vi "LoggerRefnumGetSet.vi"(8 "Logger Error In (no error)":errorcluster, 9 "menu":T2, 10 "Logger Ref Name":string, 11 "LoggerRef In":T1) -> (0 "Logger Error Out":errorcluster, 2 "refnum names":string[](array[string]), 3 "LoggerRef 2 Out":T1)   [LabVIEW 2014]
uses:
  <vilib>/Rock Robotics/WPI/Utilities/Refnum Registry Operation.ctl
  LoggerRef.ctl
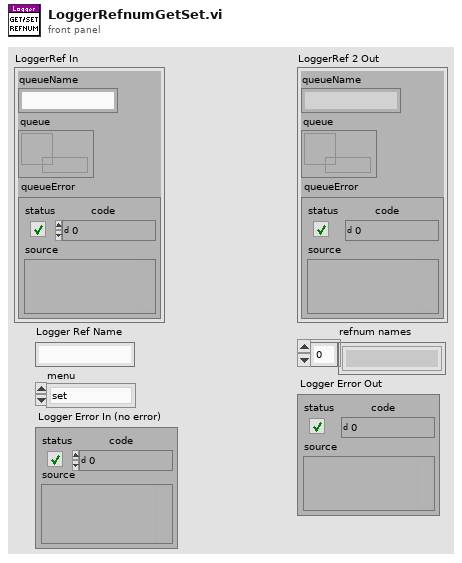
[diagram p1: front panel]
types:
  T1 = typedef "LoggerRef.ctl" = cluster{"queueName":string, "queue":refnum<queue>, "queueError":errorcluster}
  T2 = typedef "Refnum Registry Operation.ctl" = enum16{"set", "get", "delete", "get all names", "read name"}
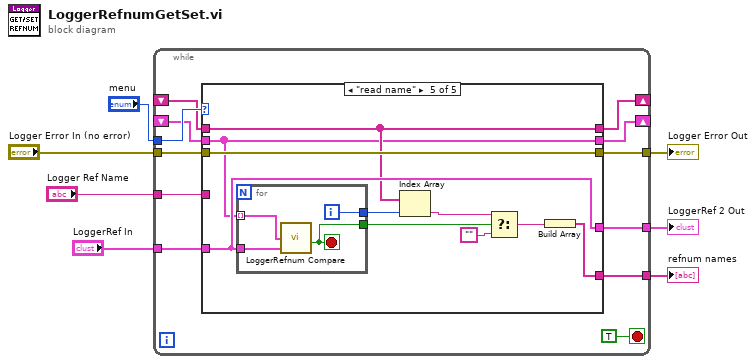
[diagram p0: block diagram]
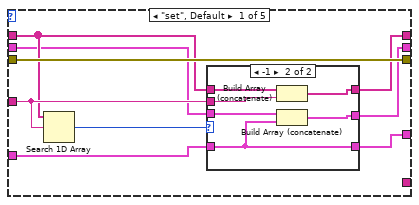
[diagram p2: hidden frame]
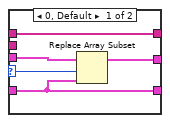
[diagram p3: hidden frame]
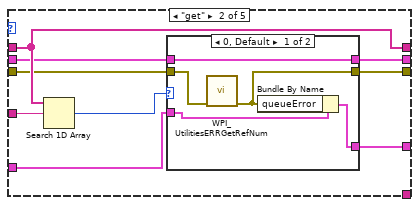
[diagram p4: hidden frame]
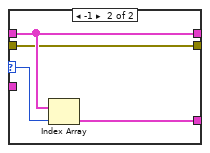
[diagram p5: hidden frame]
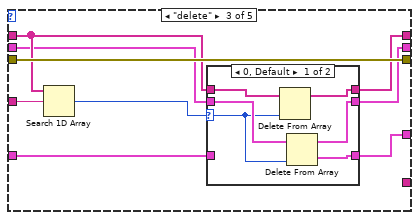
[diagram p6: hidden frame]
diagram:
  n1 = while {
    tunnel: "Logger Error In (no error)" -> [w19]
    tunnel: [w18] -> w6
    tunnel: "menu" -> [w17]
    tunnel: "LoggerRef In" -> [w16]
    shift-right: [w11] -> _
    shift-left: _ -> [w10]
    tunnel: [w15] -> w3
    tunnel: "Logger Ref Name" -> [w14]
    tunnel: [w9] -> w1
    shift-right: [w13] -> _
    shift-left: _ -> [w12]
    stop <- TRUE stop-if-true
    n2 = case shown="\"read name\"" w17 {
      tunnel: w19 -> [w28 w41 w65 w79 w89]
      tunnel: [w28 w40 w65 w79 w89] -> w18
      tunnel: w16 -> [w23 w42 w58 w78 w88]
      tunnel: [w22 w44 w59 w78 w88] -> w15
      tunnel: w14 -> [w26 w47 w66 _ _]
      tunnel: [w25 w48 w62 w76 w86] -> w13
      tunnel: w12 -> [w24 w48 w63 w76 w86]
      tunnel: [w21 w43 w60 w77 w85] -> w11
      tunnel: w10 -> [w20 w45 w61 w77 w85]
      tunnel: [_ _ _ w76 w81] -> w9
      frame "set", Default {
        n3 = Search 1D Array(1D array=w24, element=w26) -> (index of element=w27:i32)  [unwired: 1 in]
        n4 = case shown="-1" w27 {
          selector: w27 -> [w32 _]
          tunnel: w26 -> [_ w39]
          tunnel: [w29 w38] -> w25
          tunnel: w24 -> [w29 w37]
          tunnel: w23 -> [w33 w34]
          tunnel: [w33 w34] -> w22
          tunnel: [w31 w35] -> w21
          tunnel: w20 -> [w30 w36]
          frame 0, Default {
            n5 = Replace Array Subset(array=w30, new element=w33, index=w32) -> (w31:T1[])
          }
          frame -1 {
            n6 = Build Array (concatenate)(w37, w39) -> (w38:string[])
            n7 = Build Array (concatenate)(w36, w34) -> (w35:T1[])
          }
        }
      }
      frame "get" {
        n8 = Search 1D Array(1D array=w48, element=w47) -> (index of element=w46:i32)  [unwired: 1 in]
        n9 = case shown="0, Default" w46 {
          selector: w46 -> [_ w57]
          tunnel: w45 -> [w53 w55]
          tunnel: [w49 w56] -> w44
          tunnel: [w53 w55] -> w43
          tunnel: w42 -> [w51 _]
          tunnel: w41 -> [w52 w54]
          tunnel: [w50 w54] -> w40
          frame 0, Default {
            n10 = call <vilib>:"WPI_UtilitiesERRGetRefNum.vi"("error in (no error)"=w52) -> ("ERRGetRefNum"=w50:errorcluster)  [unwired: 10 out]
            n11 = Bundle By Name(cluster=w51, "queueError"=w50) -> (w49:T1)
          }
          frame -1 {
            n12 = Index Array(array=w55, index=w57) -> (element=w56:T1)
          }
        }
      }
      frame "delete" {
        n13 = Search 1D Array(1D array=w63, element=w66) -> (index of element=w64:i32)  [unwired: 1 in]
        n14 = case shown="0, Default" w64 {
          selector: w64 -> [w67 _]
          tunnel: w63 -> [w72 w75]
          tunnel: [w71 w75] -> w62
          tunnel: w61 -> [w70 w74]
          tunnel: [w69 w74] -> w60
          tunnel: [w68 w73] -> w59
          tunnel: w58 -> [_ w73]
          frame 0, Default {
            n15 = Delete From Array(array=w72, index=w67) -> (array with subset deleted=w71:string[])  [unwired: 1 in, 1 out]
            n16 = Delete From Array(array=w70, index=w67) -> (deleted portion=w68:T1, array with subset deleted=w69:T1[])  [unwired: 1 in]
          }
          frame -1 {
          }
        }
      }
      frame "get all names" {
      }
      frame "read name" {
        n17 = for {
          tunnel: w85 -> [w92] mode=indexing
          tunnel: w88 -> [w91]
          tunnel: [w93] -> w87
          tunnel: [w90] -> w83
          i -> [w93]
          stop <- w90 stop-if-true
          n18 = call "LoggerRefnum Compare.vi"("LoggerRef A"=w92, "LoggerRef B"=w91) -> ("A=B?"=w90:bool)  [unwired: 4 in]
        }
        n19 = Index Array(array=w86, index=w87) -> (element=w82:string)
        n20 = Select(t=w82, s=w83, f="") -> (s? t:f=w80:string)
        n21 = Build Array(w80) -> (w81:string[])
      }
    }
  }
  "LoggerRef 2 Out" <- w3
  "Logger Error Out" <- w6
  "refnum names" <- w1
